vi "Parse Tree Parameters.vi"(0 "Custom Device Ref":T1 format="%.0x", 1 "Rx? (T:True, F: False (Tx))":bool, 5 "Item Ref in":T1 format="%.0x", 9 "Specified Channel Ref List":T1[](array[typedef]) format="%.0x", 11 "error in":errorcluster) -> (4 "Item Ref out":T1 format="%.0x", 14 "Parameter Driver Data":T2 {"Item Refs" format="%.0x"; "Block Data Refs"."Data Reference" format="%.0x"; "Num Bits" min=1 max=32; "Start Bit" min=8 max=31}, 15 "error out":errorcluster)   [LabVIEW 2016, in "Ballard Arinc-429 System Explorer.lvlib"]
uses:
  Ballard Arinc-429 System Explorer.lvlib
  <vilib>/NI VeriStand/Custom Device API/Custom Device API.lvlib
  <vilib>/NI VeriStand/Custom Device Tools/Custom Device Utility Library/Custom Device Utility Library.lvlib
  Shared/Controls and Global/Global.vi
  Shared/Ballard Arinc-429 Shared.lvlib
  <vilib>/NI Veristand/Custom Device API/Get Item Property (I32).vi
  <vilib>/NI Veristand/Custom Device API/Get Item Property (Double).vi
  Shared/Controls and Global/Start Bit.ctl
  Shared/Controls and Global/Number of Bits.ctl
  Shared/Controls and Global/RT Param Setting.ctl
  <vilib>/NI Veristand/Custom Device API/Data Reference.ctl
  <vilib>/NI Veristand/Custom Device API/Data Access Type.ctl
  <vilib>/NI Veristand/Custom Device API/Get Item Property (Boolean).vi
  <vilib>/NI Veristand/Custom Device Tools/Custom Device Utility Library/NI VeriStand - Search for All Items by GUID.vi
  <vilib>/NI Veristand/Custom Device API/Block Data Reference.ctl
  <vilib>/NI Veristand/Custom Device API/Custom Device Item Ref.ctl
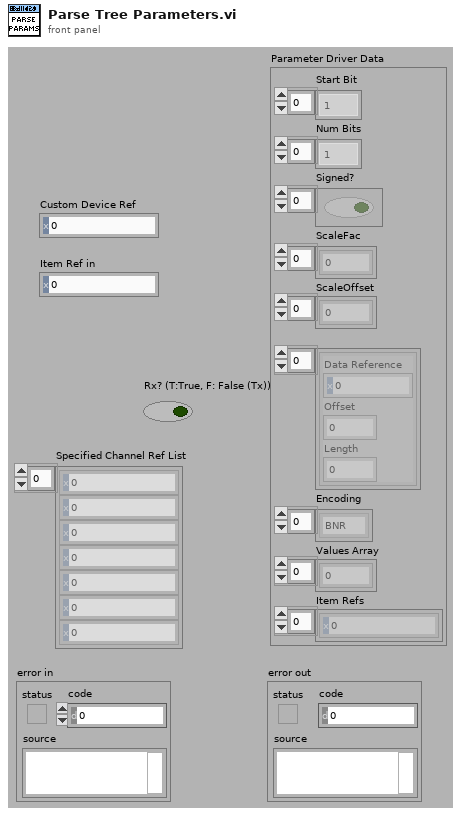
[diagram p1: front panel]
types:
  T1 = typedef "Custom Device API.lvlib/Custom Device Item Ref.ctl" = u64
  T2 = typedef "Ballard Arinc-429 Shared.lvlib/RT Param Setting.ctl" = cluster{"Start Bit":T3[], "Num Bits":T4[], "Signed?":bool[], "ScaleFac":dbl[], "ScaleOffset":dbl[], "Block Data Refs":T5[], "Encoding":enum16{"BNR", "BCD", "Discrete"}[], "Values Array":dbl[], "Item Refs":T1[]}
  T3 = typedef "Ballard Arinc-429 Shared.lvlib/Start Bit.ctl" = i32
  T4 = typedef "Ballard Arinc-429 Shared.lvlib/Number of Bits.ctl" = i32
  T5 = typedef "Custom Device API.lvlib/Block Data Reference.ctl" = cluster{"Data Reference":T6, "Offset":u64, "Length":u64}
  T6 = typedef "Custom Device API.lvlib/Data Reference.ctl" = i32
  T7 = typedef "Custom Device API.lvlib/Data Access Type.ctl" = enum16{"Read", "Write"}
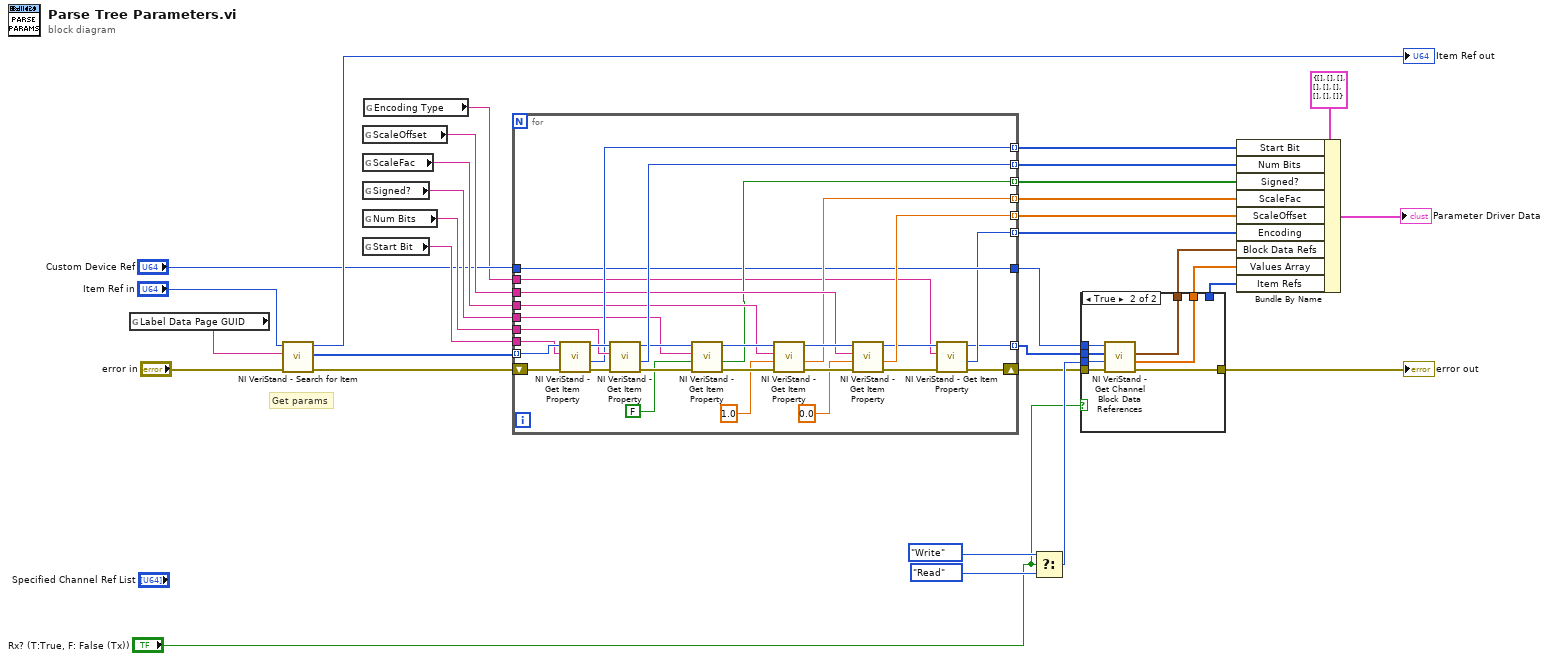
[diagram p0: block diagram]
diagram:
  # "Get params"
  n1 = global read "Global.vi" "Label Data Page GUID"() -> (w30:string)
  n2 = call-poly <vilib>:"NI VeriStand - Search for Item.vi"("error in"="error in", "Item GUID"=w30, "Section Ref in"="Item Ref in") -> ("error out"=w27:errorcluster, "Item Refs"=w26:T1[], "Section Ref out"=→"Item Ref out":T1)  [unwired: 5 in, 1 out]
  n3 = global read "Global.vi" "ScaleOffset"() -> (w20:string)
  n4 = global read "Global.vi" "ScaleFac"() -> (w21:string)
  n5 = global read "Global.vi" "Signed?"() -> (w22:string)
  n6 = global read "Global.vi" "Num Bits"() -> (w32:string)
  n7 = global read "Global.vi" "Start Bit"() -> (w31:string)
  n8 = global read "Global.vi" "Encoding Type"() -> (w13:string)
  n9 = for {
    shift-right: [w34] -> w5
    shift-left: w27 -> [w62]
    tunnel: w26 -> [w61] mode=indexing
    tunnel: w31 -> [w58]
    tunnel: w32 -> [w57]
    tunnel: [w56] -> w24 mode=indexing
    tunnel: [w55] -> w23 mode=indexing
    tunnel: w22 -> [w48]
    tunnel: w21 -> [w46]
    tunnel: w20 -> [w44]
    tunnel: [w42] -> w19 mode=indexing
    tunnel: [w41] -> w18 mode=indexing
    tunnel: [w40] -> w17 mode=indexing
    tunnel: "Custom Device Ref" -> [w39]
    tunnel: [w39] -> w9
    tunnel: w13 -> [w36]
    tunnel: [w35] -> w12 mode=indexing
    tunnel: [w33] -> w10 mode=indexing
    n10 = call-poly <vilib>:"NI VeriStand - Get Item Property.vi"("error in (no error)"=w62, "Property Name"=w58, "Item Ref in"=w61) -> ("error out"=w60:errorcluster, "Value"=w56:i32, "Item Ref out"=w59:T1)  [unwired: 5 in, 1 out]
    n11 = call-poly <vilib>:"NI VeriStand - Get Item Property.vi"("error in (no error)"=w60, "Property Name"=w57, "Item Ref in"=w59) -> ("error out"=w49:errorcluster, "Value"=w55:i32, "Item Ref out"=w54:T1)  [unwired: 5 in, 1 out]
    n12 = call-poly <vilib>:"NI VeriStand - Get Item Property.vi"("error in (no error)"=w49, "Default Value"=FALSE, "Property Name"=w48, "Item Ref in"=w54) -> ("error out"=w50:errorcluster, "Value"=w42:bool, "Item Ref out"=w53:T1)  [unwired: 4 in, 1 out]
    n13 = call-poly <vilib>:"NI VeriStand - Get Item Property.vi"("error in (no error)"=w50, "Default Value"=1.0, "Property Name"=w46, "Item Ref in"=w53) -> ("error out"=w51:errorcluster, "Value"=w41:dbl, "Item Ref out"=w52:T1)  [unwired: 4 in, 1 out]
    n14 = call-poly <vilib>:"NI VeriStand - Get Item Property.vi"("error in (no error)"=w51, "Default Value"=0.0, "Property Name"=w44, "Item Ref in"=w52) -> ("error out"=w38:errorcluster, "Value"=w40:dbl, "Item Ref out"=w37:T1)  [unwired: 4 in, 1 out]
    n15 = call-poly <vilib>:"NI VeriStand - Get Item Property.vi"("error in (no error)"=w38, "Property Name"=w36, "Item Ref in"=w37) -> ("error out"=w34:errorcluster, "Value"=w35:i32, "Item Ref out"=w33:T1)  [unwired: 5 in, 1 out]
  }
  n16 = Select(t=Data_Access_Type."Write" ("Access"), s="Rx? (T:True, F: False (Tx))", f=Data_Access_Type."Read" ("Access")) -> (s? t:f=w6:T7)
  n17 = case shown="True" "Rx? (T:True, F: False (Tx))" {
    tunnel: w10 -> [w64 w71]
    tunnel: w9 -> [_ w70]
    tunnel: [_ w69] -> w8
    tunnel: [_ w68] -> w7
    tunnel: w6 -> [_ w67]
    tunnel: w5 -> [w63 w66]
    tunnel: [w63 w65] -> w4
    tunnel: [w64 _] -> w1
    frame False {
    }
    frame True {
      n18 = call <vilib>:"NI VeriStand - Get Channel Block Data References.vi"("error in (no error)"=w66, "Access"=w67, "Channel Refs"=w71, "Device Ref in"=w70) -> ("error out"=w65:errorcluster, "Values Array"=w68:dbl[], "Block Data Refs"=w69:T5[])  [unwired: 4 in, 1 out]
    }
  }
  "error out" <- w4
  n19 = Bundle By Name(cluster=T2 {"Start Bit"=[], "Num Bits"=[], "Signed?"=[], "ScaleFac"=[], "ScaleOffset"=[], "Block Data Refs"=[], "Encoding"=[], "Values Array"=[], "Item Refs"=[]} ("Param Setting"), "Start Bit"=w24, "Num Bits"=w23, "Signed?"=w19, "ScaleFac"=w18, "ScaleOffset"=w17, "Encoding"=w12, "Block Data Refs"=w8, "Values Array"=w7, "Item Refs"=w1) -> (→"Parameter Driver Data":T2)
